vi "master_python_v2.0.vi"() -> ()   [LabVIEW 2026]
uses:
  <vilib>/Utility/error.llb/DialogType.ctl
  <vilib>/DAQmx/write.llb/DAQmx Write (Analog 2D DBL NChan NSamp).vi
  <vilib>/DAQmx/read.llb/DAQmx Read (Analog 1D Wfm NChan NSamp).vi
  <vilib>/DAQmx/miscellaneous.llb/DAQmx Fill In Error Info.vi
  <vilib>/Utility/inputDevices.llb/keyboardAcquire.vi
  Nanostage/Madlib.dll
panel:
  out "QPD":dbl
  out "Pos 0":dbl
  in  "Comment":string
  out "loop iteration":i32
  out "x start":dbl
  out "y start":dbl
  out "z start":dbl
  out "start iteration":dbl
  out "data":waveform(dbl)[](array[waveform])
  out "Numeric 2":i32
  out "Numeric":i32
  out "stop Ind":bool
  in  "Tab Control":enum32{"Main Control", "Calibration"}(tab)
  in  "Apply Force":bool
  out "Waveform Chart 6":waveform(dbl)(graph)
  out "Waveform Chart 5":waveform(dbl)(graph)
  in  "stop":bool
  in  "Record Data":bool
  in  "New File?":bool caption="new_file"
  out "QPD Position":cluster{"Array":dbl[], "Array":dbl[]}(graph)
  out "MT channels":waveform(dbl)[](graph)
  out "QPD Precise Position":cluster{"Array":dbl[], "Array":dbl[]}(graph)
  out "QPD Sum (Volt)":waveform(dbl)(graph)
  out "x":dbl
  out "y":dbl
  out "z":dbl
  in  "<":bool
  in  ">":bool
  in  "v":bool
  in  "^":bool
  in  "Down":bool
  in  "Up":bool
  in  "Fine":dbl=50.0
  in  "Step Size (nm)":bool
  in  "Course":dbl=500.0
  in  "Enable\ntapping":bool
  in  "DELAY (ms)":u32=10
  in  "x amplitude\n(um)":dbl
  in  "speed":i32=1
  in  "z amplitude (um)":dbl
  out "# oscillations":dbl
  in  "y amplitude\n(um)":dbl min=-25.0 max=25.0 step=0.05
  in  "Samples":u16=100 min=1 step=1
  in  "Centre":bool
  in  "Power Spectrum":bool
  in  "Duration (s)":dbl=2.0
  in  "Boolean":bool
  in  "Frequency":dbl=1.0 min=0.0 max=100.0 step=0.01
  in  "Amplitude":dbl=0.5 min=0.1 max=0.9 step=0.1
  in  "# Cycles":dbl=50.0 min=0.0 max=10000.0 step=0.001
  in  "Start Signal\nGen":bool
  in  "Desired Force (pN)":dbl step=0.01
  out "Measured Force (pN)":dbl(slide) scale=-2.0..2.0
  in  "Save Spectrum":bool
  in  "#":i32=1
  out "QPD nLR":waveform(dbl)(graph)
  out "QPD nBT":waveform(dbl)(graph)
  in  "Filename":path=path "C:/Users/localadmin/Desktop/220601 beadscan/7umscan2umbead.lvm"
  in  "Set 0 pN Position":bool
  out "QPD0":dbl
  in  "reinitialize?":bool
  in  "Conversion factor (pN/V)":dbl=1.0
  # "Left= anticlockwise"
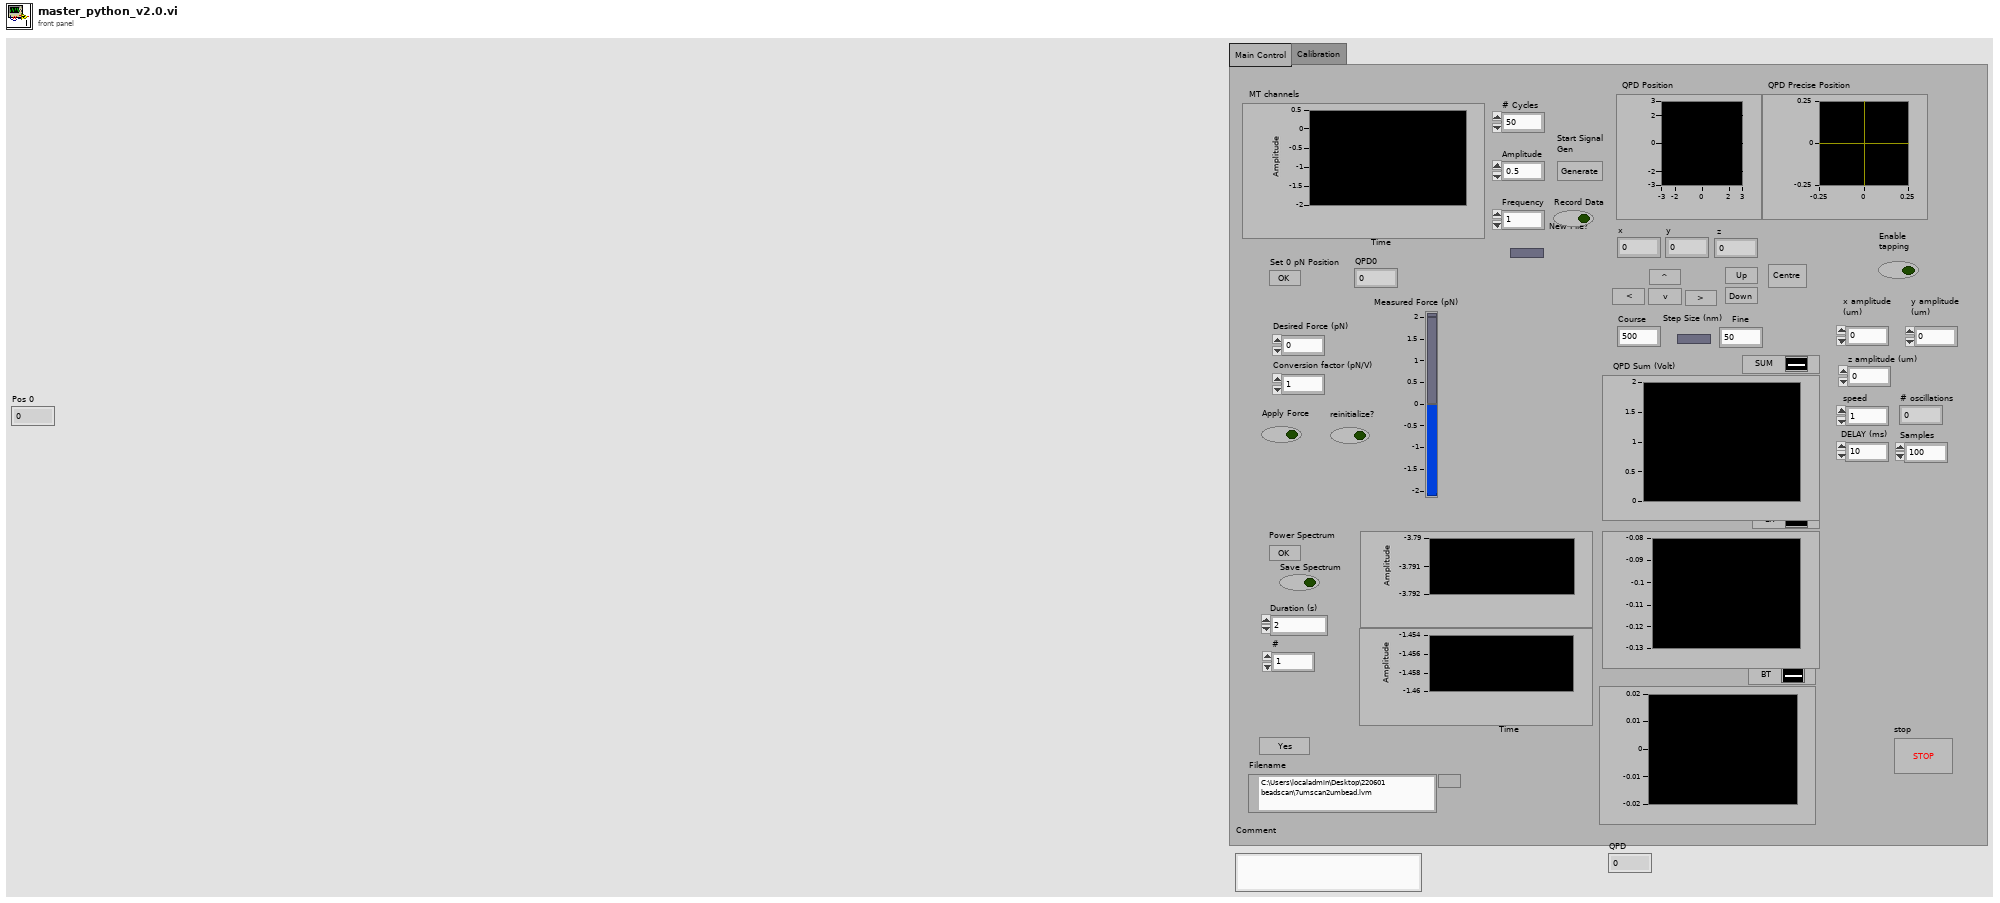
[diagram p1: front panel]
types:
  T1 = typedef "DialogType.ctl" = u16
  T2 = enum16{"Centre", "Move", "Tapping", "Calibration"}
  T3 = enum16{"0", "1", "2", "3", "4", "5", "6", "7", "8", "9", "A", "B", "C", "D", "E", "F", "G", "H", "I", "J", "K", "L", "M", "N", "O", "P", "Q", "R", "S", "T", "U", "V", "W", "X", "Y", "Z", "F1", "F2", "F3", "F4", "F5", "F6", "F7", "F8", "F9", "F10", "F11", "F12", "F13", "F14", "F15", "ADD", "BACK", "BACKSLASH", "CAPITAL", "COMMA", "DECIMAL", "DELETE", "DIVIDE", "DOWN", "END", "EQUALS", "ESCAPE", "GRAVE (`)", "HOME", "INSERT", "LBRACKET", "LCONTROL", "LEFT", "L ALT", "LSHIFT", "LWIN", "MINUS", "MULTIPLY", "NEXT", "NUMLOCK", "NUMPAD_0", "NUMPAD_1", "NUMPAD_2", "NUMPAD_3", "NUMPAD_4", "NUMPAD_5", "NUMPAD_6", "NUMPAD_7", "NUMPAD_8", "NUMPAD_9", "PAUSE", "PERIOD", "PRIOR (PG UP)", "RBRACKET", "RCONTROL", "RETURN", "RIGHT", "R ALT", "RSHIFT", "RWIN", "SCROLL", "SEMICOLON", "SLASH", "SPACE", "SUBTRACT", "TAB", "UP", "ENTER (num pad)", "' (quote)"}[]
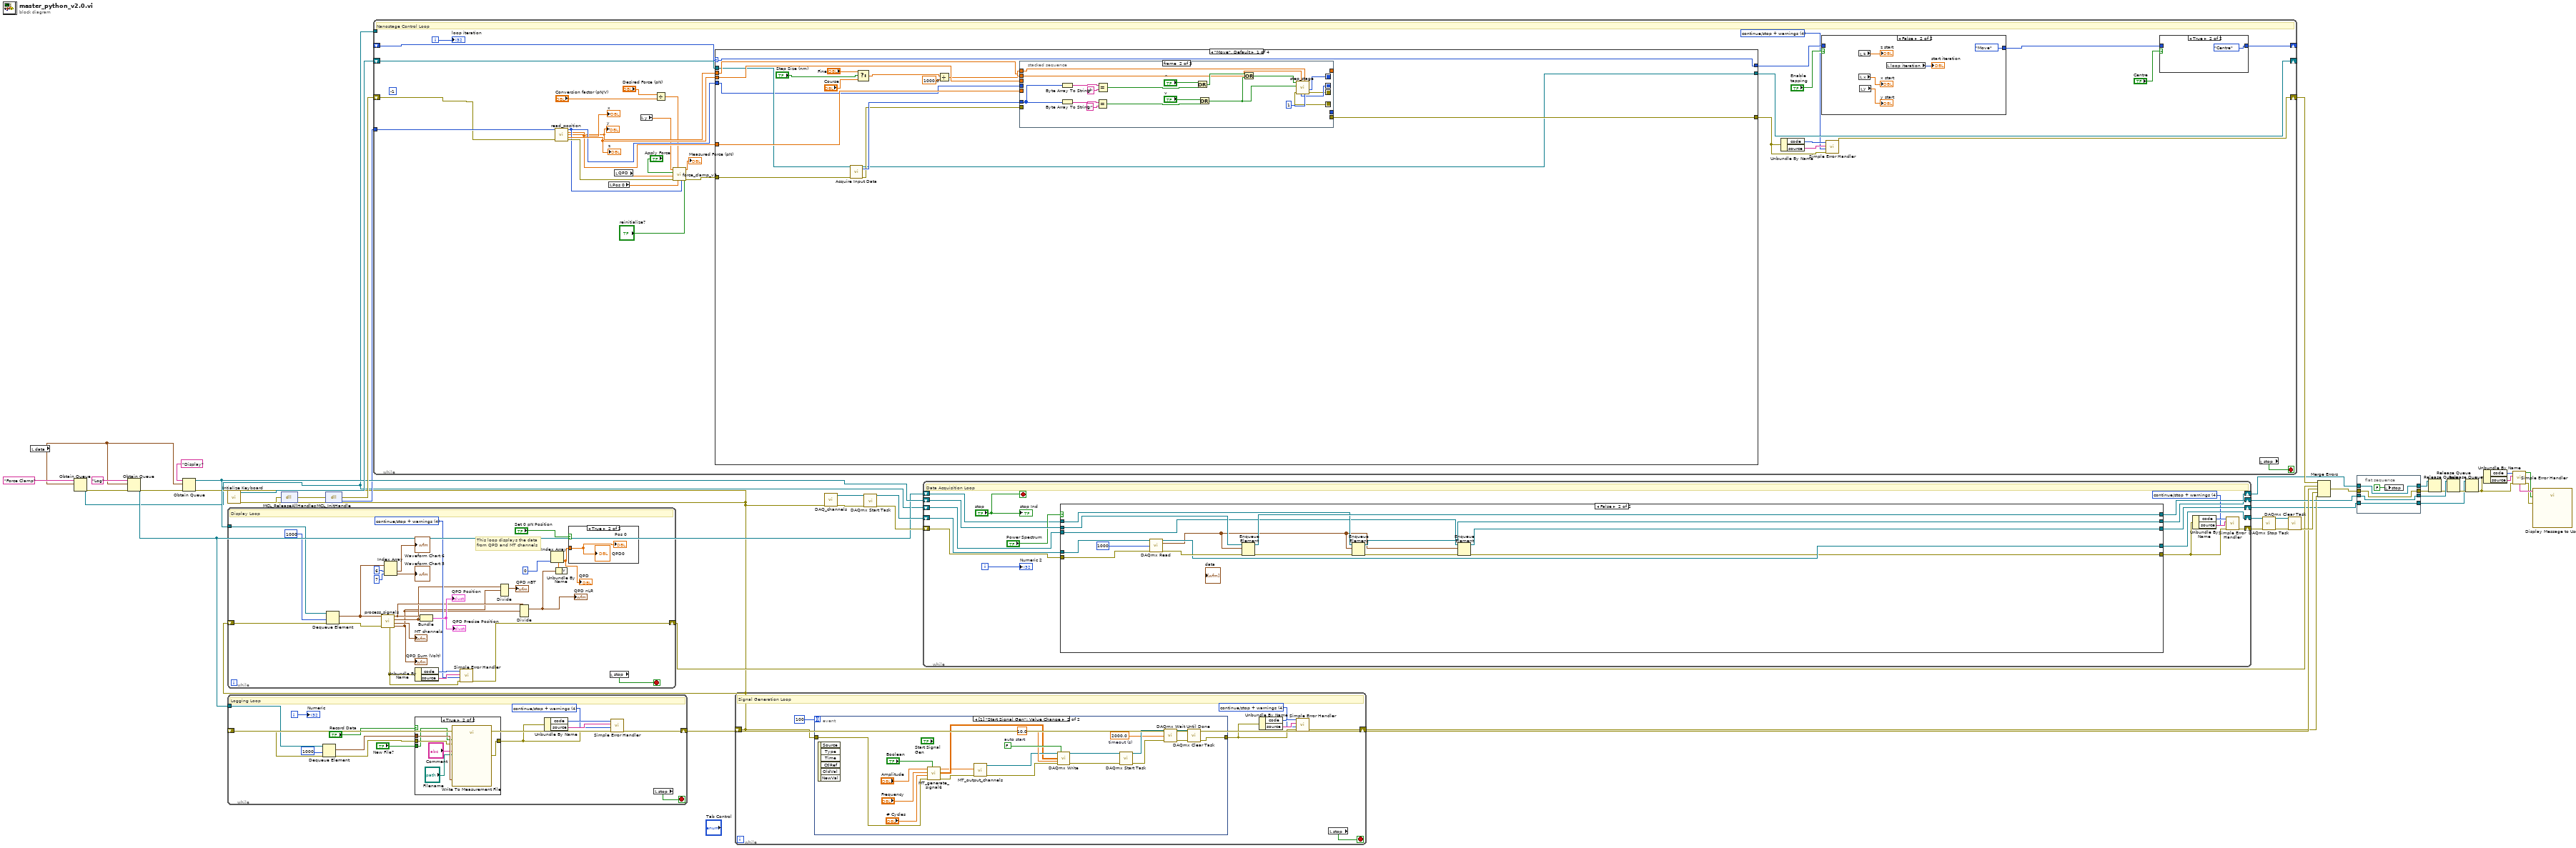
[diagram p0: block diagram]
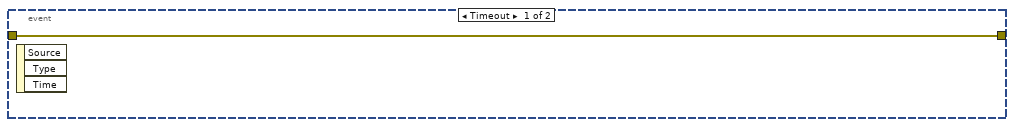
[diagram p2: hidden frame]
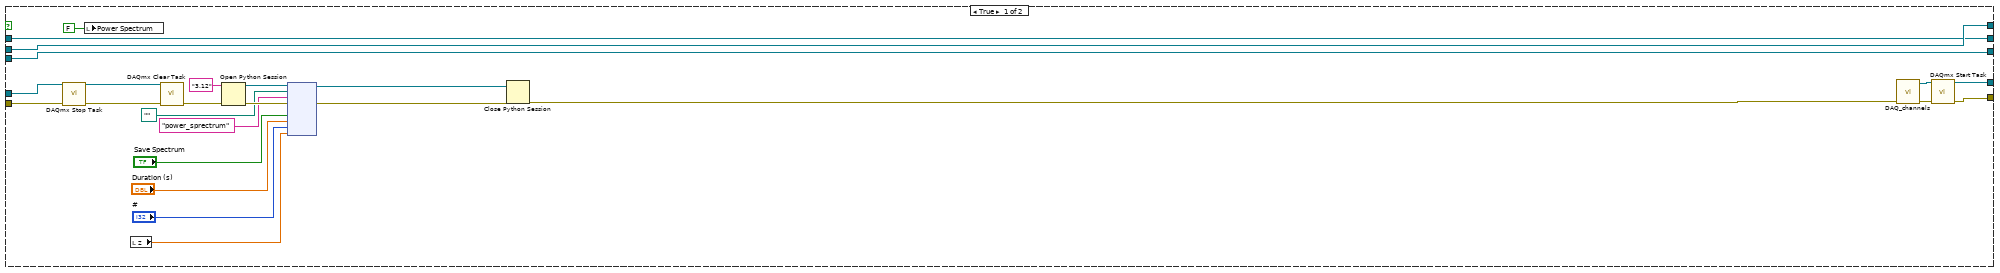
[diagram p3: hidden frame]
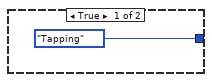
[diagram p6: hidden frame]
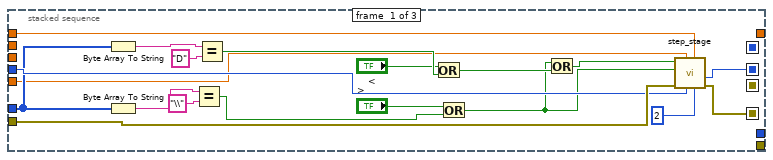
[diagram p7: hidden frame]
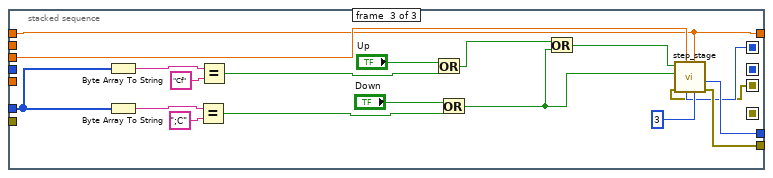
[diagram p8: hidden frame]
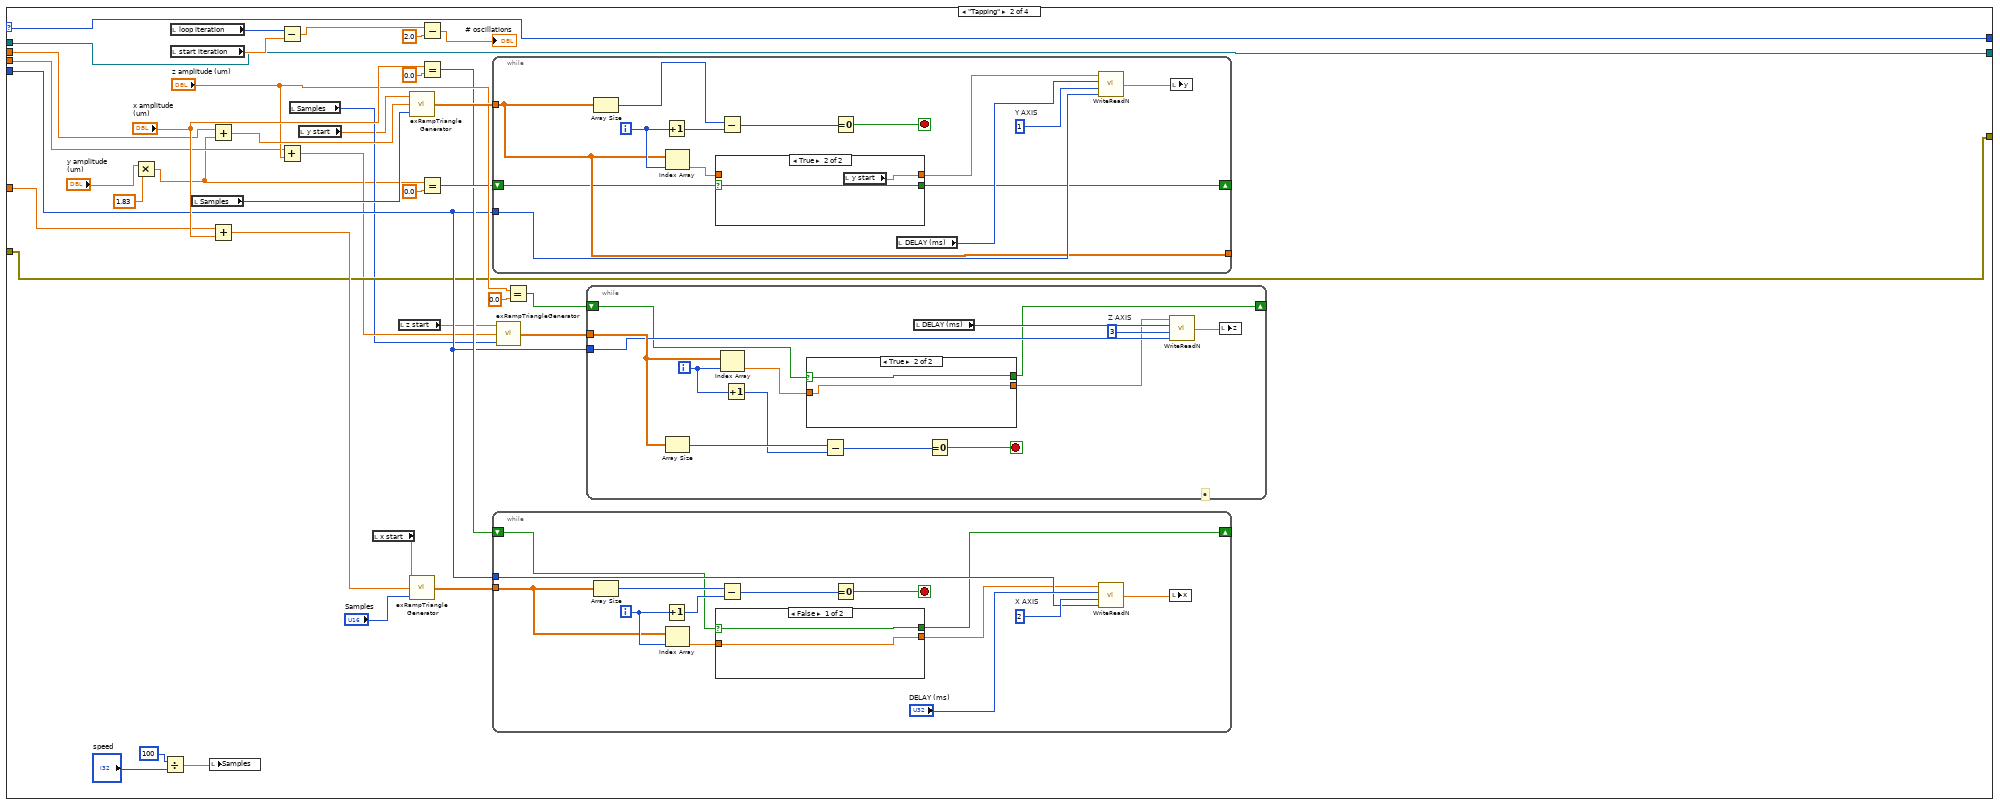
[diagram p9: hidden frame]
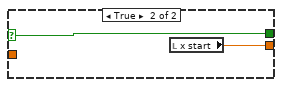
[diagram p12: hidden frame]
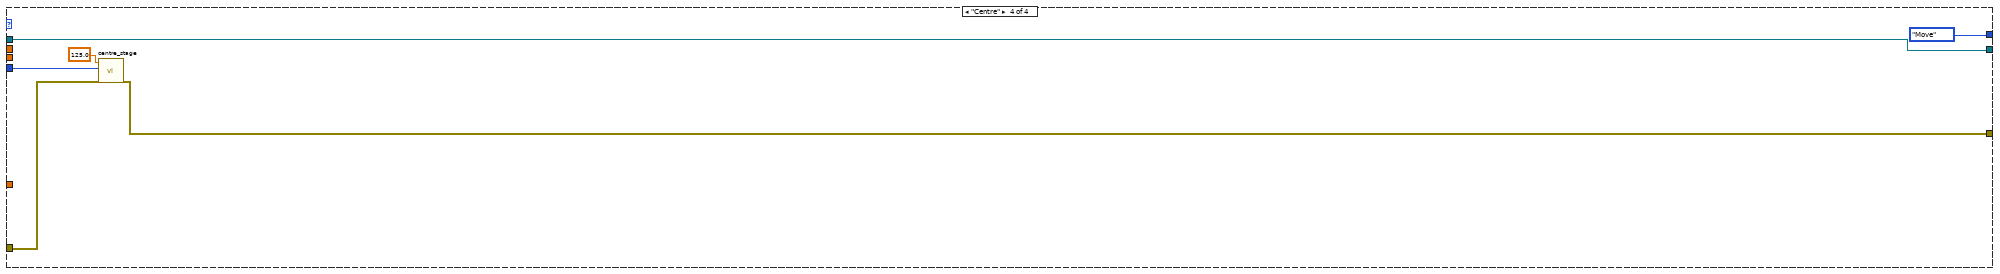
[diagram p14: hidden frame]
diagram:
  n1 = local read "data"() -> (w6:waveform(dbl)[])
  n2 = Obtain Queue(name (unnamed)="Force Clamp", element data type=w6) -> (queue out=w1:refnum<queue>, error out=w8:errorcluster)  [unwired: 3 in, 1 out]
  n3 = Obtain Queue(name (unnamed)="Log", element data type=w6, error in (no error)=w8) -> (queue out=w12:refnum<queue>, error out=w17:errorcluster)  [unwired: 2 in, 1 out]
  n4 = Obtain Queue(name (unnamed)="Display", element data type=w6, error in (no error)=w17) -> (queue out=w19:refnum<queue>, error out=w10:errorcluster)  [unwired: 2 in, 1 out]
  n5 = call <vilib>:"Intialize Keyboard.vi"("error in (no error)"=w10) -> ("error out"=w23:errorcluster, "device ID"=w21:refnum<k1>)  [unwired: 9 out]
  n6 = while {
    tunnel: w19 -> [w70]
    shift-right: [w55] -> w26
    shift-left: w10 -> [w69]
    stop <- w68 stop-if-true
    w54 = T1 4 items=["no dialog", "OK message", "continue or stop message", "OK message + warnings", "continue/stop + warnings"] ("type of dialog (OK msg:1)")
    # "This loop displays the data from QPD and MT channels"
    # "Display Loop"
    n7 = Dequeue Element(queue=w70, timeout in ms (-1)=1000, error in (no error)=w69) -> (element=w60:waveform(dbl)[], error out=w62:errorcluster)  [unwired: 2 out]
    n8 = call "process_signals.vi"("error in (no error)"=w62, "data"=w60) -> ("SUM"=w50:waveform(dbl), "MT"=→"MT channels":waveform(dbl)[], "BT"=w51:waveform(dbl), "LR"=w52:waveform(dbl), "error out"=w63:errorcluster)  [unwired: 5 in]
    "QPD Sum (Volt)" <- w50
    n9 = Index Array(array=w60, index #1=6 ("index"), index #2=7 ("index")) -> (element #1=→"Waveform Chart 6":waveform(dbl), element #2=→"Waveform Chart 5":waveform(dbl))
    n10 = Unbundle By Name(w63) -> ("code"=w65:i32, "source"=w64:string)
    n11 = Bundle("LR"=w52, "BT"=w51) -> (→"QPD Position" →"QPD Precise Position":cluster{"LR":waveform(dbl), "BT":waveform(dbl)})  [unwired: 1 in]
    n12 = call <vilib>:"Simple Error Handler.vi"("error code (no error:0)"=w65, "error source (\" \")"=w64, "type of dialog (OK msg:1)"=w54, "error in (no error)"=w63) -> ("error out"=w55:errorcluster)  [unwired: 1 in, 4 out]
    n13 = Divide(1:w50, 2:w51) -> (0:→"QPD nBT":waveform(dbl))  [unwired: 1 in, 1 out]
    n14 = Divide(1:w50, 2:w52) -> (0:w47:waveform(dbl))  [unwired: 1 in, 1 out]
    "QPD nLR" <- w47
    n15 = Unbundle By Name(w47) -> ("Y"=w48:dbl[])
    n16 = Index Array(array=w48, index=0) -> (element=w45:dbl)
    "QPD" <- w45
    n17 = case shown="True" "Set 0 pN Position" {
      tunnel: w45 -> [_ w71]
      frame False {
      }
      frame True {
        "Pos 0" <- w71
        "QPD0" <- w71
      }
    }
    n18 = local read "stop"() -> (w68:bool)
  }
  n19 = while {
    shift-right: [w73] -> w30
    shift-left: w10 -> [w85]
    tunnel: w12 -> [w84]
    i -> [w79]
    stop <- w74 stop-if-true
    w72 = T1 4 items=["no dialog", "OK message", "continue or stop message", "OK message + warnings", "continue/stop + warnings"] ("type of dialog (OK msg:1)")
    # "Logging Loop"
    n20 = Dequeue Element(queue=w84, timeout in ms (-1)=1000, error in (no error)=w85) -> (element=w81:waveform(dbl)[], error out=w82:errorcluster)  [unwired: 2 out]
    n21 = case shown="True" "Record Data" {
      tunnel: [w86 w92] -> w75
      tunnel: w81 -> [_ w91]
      tunnel: "New File?" -> [_ w88]
      tunnel: w82 -> [w86 w90]
      frame False {
      }
      frame True {
        n22 = call "Write To Measurement File"("Signals"=w91, "new_file"=w88, "error in (no error)"=w90, "Filename"="Filename", "Comment"="Comment") -> ("error out"=w92:errorcluster)  [unwired: 12 in, 2 out]
      }
    }
    n23 = Unbundle By Name(w75) -> ("code"=w77:i32, "source"=w76:string)
    n24 = call <vilib>:"Simple Error Handler.vi"("error code (no error:0)"=w77, "error source (\" \")"=w76, "type of dialog (OK msg:1)"=w72, "error in (no error)"=w75) -> ("error out"=w73:errorcluster)  [unwired: 1 in, 4 out]
    n25 = local read "stop"() -> (w74:bool)
    "Numeric" <- w79
  }
  n26 = dll-call lib="C:/Users/psmr500/PycharmProjects/COMBI-Tweez/LabVIEW Microscope Control/Nanostage/MADLib.dll" fn="MCL_ReleaseAllHandles"(error in=w23) -> (error out=w24:errorcluster)  [unwired: 3 in, 1 out]
  n27 = dll-call lib="C:/Users/psmr500/PycharmProjects/COMBI-Tweez/LabVIEW Microscope Control/Nanostage/MADLib.dll" fn="MCL_InitHandle"(error in=w24) -> (error out=w22:errorcluster, "return type"=w11:i32)  [unwired: 2 in, 1 out]
  n28 = while {
    shift-right: [w106] -> w20
    shift-left: w22 -> [w101]
    shift-right: [w117] -> _
    shift-left: w21 -> [w119]
    shift-right: [w111] -> _
    shift-left: _ -> [w118]
    tunnel: w11 -> [w116]
    tunnel: w1 -> [_]
    i -> [w114]
    stop <- w124 stop-if-true
    (unwired) -1 ("timeout in ms (-1)")
    w105 = T1 4 items=["no dialog", "OK message", "continue or stop message", "OK message + warnings", "continue/stop + warnings"] ("type of dialog (OK msg:1)")
    # "Nanostage Control Loop"
    n29 = call "read_position.vi"("handle in"=w116, "error in (no error)"=w101) -> ("handle out"=w107:i32, "x"=w104:dbl, "y"=w103:dbl, "z"=w120:dbl, "error out"=w109:errorcluster)  [unwired: 9 in]
    "x" <- w104
    "y" <- w103
    "z" <- w120
    n30 = local read "Pos 0"() -> (w98:dbl)
    n31 = local read "QPD"() -> (w99:dbl)
    n32 = local read "y"() -> (w100:dbl)
    n33 = Divide(x="Desired Force (pN)", y="Conversion factor (pN/V)") -> (x/y=w95:dbl)
    n34 = call "force_clamp_v3.vi"("reinitialize? (F) 2"="reinitialize?", "handle in"=w107, "Pos 0"=w98, "Desired Force (pN)"=w95, "error in (no error)"=w109, "QPD"=w99, "Apply Force"="Apply Force", "Nanostage"=w100) -> ("error out"=w108:errorcluster, "QPD delta"=→"Measured Force (pN)":dbl)  [unwired: 2 in]
    n35 = case shown="\"Move\", Default" w118 {
      selector: w118 -> [w133 w217 w308 _]
      tunnel: w108 -> [w139 w219 w306 w323]
      tunnel: w107 -> [w137 w220 w307 w322]
      tunnel: [w135 w219 w300 w321] -> w121
      tunnel: w104 -> [w149 w222 w310 _]
      tunnel: w103 -> [w148 w221 w309 _]
      tunnel: w120 -> [w147 w216 _ _]
      tunnel: w119 -> [w140 w218 w299 w318]
      tunnel: [w133 w217 w308 T2."Move"] -> w115
      tunnel: [w134 w218 w299 w318] -> w117
      frame "Move", Default {
        n36 = call-poly <vilib>:"Acquire Input Data.vi"("device ID"=w140, "error in (no error)"=w139) -> ("device ID"=w134:refnum<k1>, "keys pressed"=w138:T3, "error out"=w136:errorcluster)  [unwired: 15 out]
        n37 = Select(t="Fine", s="Step Size (nm)", f="Course") -> (s? t:f=w143:dbl)
        n38 = Divide(x=w143, y=1000.0) -> (x/y=w141:dbl)
        n39 = stacked-sequence {
          seq-local: [w165 _ _] -> [_ w185 _]
          seq-local: [w164 _ _] -> [_ w184 _]
          seq-local: [_ w182 _] -> [_ _ w202]
          seq-local: [_ w183 _] -> [_ _ w201]
          tunnel: w136 -> [w168 _ _]
          tunnel: w137 -> [w167 _ _]
          tunnel: w149 -> [w151 _ _]
          tunnel: w148 -> [_ w169 _]
          tunnel: w147 -> [_ _ w205]
          tunnel: [_ _ w203] -> w135
          tunnel: [_ _ w204] -> _
          tunnel: w138 -> [w153 w171 w189]
          tunnel: [_ _ w188] -> _
          tunnel: w141 -> [w152 w170 w188]
          frame #0 {
            n40 = Byte Array To String(unsigned byte array=w153) -> (string=w161:string)
            n41 = Byte Array To String(unsigned byte array=w153) -> (string=w163:string)
            n42 = Equal?(x=w163, y="\\") -> (x = y?=w159:bool)
            n43 = Equal?(x=w161, y="D") -> (x = y?=w158:bool)
            n44 = Or(x="<", y=w158) -> (x .or. y?=w155:bool)
            n45 = Or(x=">", y=w159) -> (x .or. y?=w150:bool)
            n46 = Or(x=w150, y=w155) -> (x .or. y?=w154:bool)
            n47 = call "step_stage.vi"("axis"=u32 2, "step"=w152, "handle"=w167, "position"=w151, "error in"=w168, "+/-"=w150, "move"=w154) -> ("error out"=w164:errorcluster, "handle out"=w165:i32)  [unwired: 3 in]
          }
          frame #1 {
            n48 = Byte Array To String(unsigned byte array=w171) -> (string=w181:string)
            n49 = Byte Array To String(unsigned byte array=w171) -> (string=w179:string)
            n50 = Equal?(x=w179, y=";") -> (x = y?=w174:bool)
            n51 = Equal?(x=w181, y="f") -> (x = y?=w177:bool)
            n52 = Or(x="^", y=w177) -> (x .or. y?=w173:bool)
            n53 = Or(x="v", y=w174) -> (x .or. y?=w172:bool)
            n54 = Or(x=w173, y=w172) -> (x .or. y?=w187:bool)
            n55 = call "step_stage.vi"("axis"=u32 1, "step"=w170, "handle"=w185, "position"=w169, "error in"=w184, "+/-"=w172, "move"=w187) -> ("error out"=w183:errorcluster, "handle out"=w182:i32)  [unwired: 3 in]
          }
          frame #2 {
            n56 = Byte Array To String(unsigned byte array=w189) -> (string=w200:string)
            n57 = Byte Array To String(unsigned byte array=w189) -> (string=w198:string)
            n58 = Equal?(x=w198, y=";C") -> (x = y?=w195:bool)
            n59 = Equal?(x=w200, y="Cf") -> (x = y?=w196:bool)
            n60 = Or(x="Up", y=w196) -> (x .or. y?=w194:bool)
            n61 = Or(x="Down", y=w195) -> (x .or. y?=w192:bool)
            n62 = Or(x=w194, y=w192) -> (x .or. y?=w193:bool)
            n63 = call "step_stage.vi"("axis"=u32 3, "step"=w188, "handle"=w202, "position"=w205, "error in"=w201, "+/-"=w192, "move"=w193) -> ("error out"=w203:errorcluster, "handle out"=w204:i32)  [unwired: 3 in]
          }
        }
      }
      frame "Tapping" {
        n64 = Multiply(x="y amplitude\n(um)", y=1.83) -> (x*y=w208:dbl)
        n65 = Divide(x=100, y="speed") -> (x/y=w239:dbl)
        n66 = local read "loop iteration"() -> (w234:i32)
        n67 = local read "start iteration"() -> (w235:dbl)
        n68 = local read "Samples"() -> (w236:u16)
        n69 = local write "Samples"(w239) -> ()
        n70 = Add(x=w221, y=w208) -> (x+y=w238:dbl)
        n71 = Add(x=w222, y="x amplitude\n(um)") -> (x+y=w243:dbl)
        n72 = Subtract(x=w234, y=w235) -> (x-y=w233:dbl)
        n73 = Add(x=w216, y="z amplitude (um)") -> (x+y=w215:dbl)
        n74 = local read "Samples"() -> (w214:u16)
        n75 = local read "y start"() -> (w210:dbl)
        n76 = local read "x start"() -> (w212:dbl)
        n77 = local read "z start"() -> (w211:dbl)
        n78 = call "exRampTriangleGenerator.vi"("Number of positions"=w236, "End(um)"=w238, "Start(um)"=w210) -> ("Array"=w237:dbl[])
        n79 = call "exRampTriangleGenerator.vi"("Number of positions"="Samples", "End(um)"=w243, "Start(um)"=w212) -> ("Array"=w244:dbl[])
        n80 = Subtract(x=w233, y=2.0) -> (x-y=→"# oscillations":dbl)
        n81 = Equal?(x="x amplitude\n(um)", y=0.0) -> (x = y?=w224:bool)
        n82 = Equal?(x=w208, y=0.0) -> (x = y?=w225:bool)
        n83 = while {
          tunnel: [w268] -> _
          tunnel: w220 -> [w275]
          tunnel: w237 -> [w268]
          shift-right: [w264] -> _
          shift-left: w225 -> [w265]
          i -> [w276]
          stop <- w270 stop-if-true
          w271 = 1  # Y AXIS
          n84 = Array Size(array=w268) -> (size(s)=w273:i32)
          n85 = Increment(x=w276) -> (x+1=w272:i32)
          n86 = Index Array(array=w268, index=w276) -> (element=w267:dbl)
          n87 = case shown="True" w265 {
            selector: w265 -> [w277 w280]
            tunnel: w267 -> [w278 _]
            tunnel: [w278 w279] -> w266
            tunnel: [w277 w280] -> w264
            frame False {
            }
            frame True {
              n88 = local read "y start"() -> (w279:dbl)
            }
          }
          n89 = Subtract(x=w273, y=w272) -> (x-y=w274:i32)
          n90 = Equal To 0?(x=w274) -> (x = 0?=w270:bool)
          n91 = local read "DELAY (ms)"() -> (w269:u32)
          n92 = call "WriteReadN.vi"("Handle"=w275, "Axis"=w271, "Delay (ms)"=w269, "Move to (um)"=w266) -> ("Current Position (um)"=w263:dbl)
          n93 = local write "y"(w263) -> ()
        }
        n94 = while {
          tunnel: w244 -> [w286]
          tunnel: w220 -> [w287]
          shift-right: [w282] -> _
          shift-left: w224 -> [w283]
          i -> [w290]
          stop <- w292 stop-if-true
          w288 = 2  # X AXIS
          n95 = Array Size(array=w286) -> (size(s)=w293:i32)
          n96 = Increment(x=w290) -> (x+1=w291:i32)
          n97 = Index Array(array=w286, index=w290) -> (element=w285:dbl)
          n98 = case shown="False" w283 {
            selector: w283 -> [w295 w298]
            tunnel: w285 -> [w296 _]
            tunnel: [w296 w297] -> w284
            tunnel: [w295 w298] -> w282
            frame False {
            }
            frame True {
              n99 = local read "x start"() -> (w297:dbl)
            }
          }
          n100 = Subtract(x=w293, y=w291) -> (x-y=w294:i32)
          n101 = Equal To 0?(x=w294) -> (x = 0?=w292:bool)
          n102 = call "WriteReadN.vi"("Handle"=w287, "Axis"=w288, "Delay (ms)"="DELAY (ms)", "Move to (um)"=w284) -> ("Current Position (um)"=w281:dbl)
          n103 = local write "x"(w281) -> ()
        }
        n104 = call "exRampTriangleGenerator.vi"("Number of positions"=w214, "End(um)"=w215, "Start(um)"=w211) -> ("Array"=w213:dbl[])
        n105 = Equal?(x="z amplitude (um)", y=0.0) -> (x = y?=w223:bool)
        n106 = while {
          tunnel: w213 -> [w251]
          tunnel: w220 -> [w250]
          shift-right: [w246] -> _
          shift-left: w223 -> [w247]
          i -> [w254]
          stop <- w256 stop-if-true
          w253 = 3  # Z AXIS
          # "e"
          n107 = Array Size(array=w251) -> (size(s)=w257:i32)
          n108 = Index Array(array=w251, index=w254) -> (element=w249:dbl)
          n109 = Increment(x=w254) -> (x+1=w255:i32)
          n110 = case shown="True" w247 {
            selector: w247 -> [w259 w262]
            tunnel: w249 -> [w260 w261]
            tunnel: [w260 w261] -> w248
            tunnel: [w259 w262] -> w246
            frame False {
            }
            frame True {
            }
          }
          n111 = Subtract(x=w257, y=w255) -> (x-y=w258:i32)
          n112 = local read "DELAY (ms)"() -> (w252:u32)
          n113 = Equal To 0?(x=w258) -> (x = 0?=w256:bool)
          n114 = call "WriteReadN.vi"("Handle"=w250, "Axis"=w253, "Delay (ms)"=w252, "Move to (um)"=w248) -> ("Current Position (um)"=w245:dbl)
          n115 = local write "z"(w245) -> ()
        }
      }
      frame "Calibration" {
        n116 = flat-sequence {
          tunnel: w306 -> [w311]
          tunnel: [w311] -> w301
          tunnel: [w312] -> w302
          tunnel: w301 -> [w312]
          tunnel: w307 -> [_]
          tunnel: w310 -> [_]
          tunnel: w309 -> [_]
          tunnel: [w313] -> w303
          tunnel: w302 -> [w313]
          tunnel: [w314] -> w304
          tunnel: w303 -> [w314]
          tunnel: [w316] -> _
          tunnel: w307 -> [w316]
          tunnel: [w315] -> w305
          tunnel: w304 -> [w315]
          tunnel: w305 -> [w317]
          tunnel: [w317] -> w300
          frame #0 {
          }
          frame #1 {
          }
          frame #2 {
          }
          frame #3 {
          }
          frame #4 {
          }
          frame #5 {
          }
        }
      }
      frame "Centre" {
        n117 = call "centre_stage.vi"("error in"=w323, "handle in"=w322, "Destination"=125.0) -> ("error out"=w321:errorcluster)  [unwired: 7 in, 1 out]
      }
    }
    n118 = Unbundle By Name(w121) -> ("code"=w123:i32, "source"=w122:string)
    n119 = case shown="False" "Enable\ntapping" {
      tunnel: w115 -> [_ _]
      tunnel: [T2."Tapping" T2."Move"] -> w102
      frame True {
      }
      frame False {
        n120 = local read "z"() -> (→"z start":dbl)
        n121 = local read "x"() -> (→"x start":dbl)
        n122 = local read "y"() -> (→"y start":dbl)
        n123 = local read "loop iteration"() -> (→"start iteration":i32)
      }
    }
    n124 = call <vilib>:"Simple Error Handler.vi"("error code (no error:0)"=w123, "error source (\" \")"=w122, "type of dialog (OK msg:1)"=w105, "error in (no error)"=w121) -> ("error out"=w106:errorcluster)  [unwired: 1 in, 4 out]
    n125 = case shown="True" "Centre" {
      tunnel: [w125 T2."Centre"] -> w111
      tunnel: w102 -> [w125 _]
      frame False {
      }
      frame True {
      }
    }
    n126 = local read "stop"() -> (w124:bool)
    "loop iteration" <- w114
  }
  n127 = while {
    shift-right: [w325] -> w9
    shift-left: w10 -> [w330]
    stop <- w331 stop-if-true
    w326 = T1 4 items=["no dialog", "OK message", "continue or stop message", "OK message + warnings", "continue/stop + warnings"] ("type of dialog (OK msg:1)")
    # "Signal Generation Loop"
    n128 = event shown="[1] \"Start Signal Gen\": Value Change" {
      selector: _ -> [_ _]
      dyn-events: _ -> [_ _]
      timeout: 100 -> [_ _]
      tunnel: [w332 w335] -> w324
      tunnel: w330 -> [w332 w334]
      event Timeout {
        n129 = event-data() -> ()  [unwired: 1 in, 3 out]
      }
      event "Start Signal\nGen": Value Change {
        w344 = 2000.0  # timeout (s)
        w343 = FALSE  # auto start
        n130 = event-data() -> ()  [unwired: 1 in, 6 out]
        n131 = call "MT_generate_signal6.vi"("Direction"="Boolean", "error in (no error)"=w334, "# cycles"="# Cycles", "frequency"="Frequency", "amplitude"="Amplitude") -> ("error out"=w340:errorcluster, "signals out"=w338:dbl[][], "# samples"=w337:dbl)  [unwired: 4 in]
        n132 = call "MT_output_channels.vi"("error in"=w340, "number of samples"=w337) -> ("error out"=w339:errorcluster, "task out"=w341:refnum<k21>)  [unwired: 8 in]
        n133 = call-poly <vilib>:"DAQmx Write.vi"("task/channels in"=w341, "auto start"=w343, "data"=w338, "timeout"=10.0, "error in"=w339) -> ("task out"=w348:refnum<k21>, "error out"=w349:errorcluster)  [unwired: 8 in, 1 out]
        n134 = call <vilib>:"DAQmx Start Task.vi"("task/channels in"=w348, "error in"=w349) -> ("task out"=w345:refnum<k21>, "error out"=w346:errorcluster)  [unwired: 12 in]
        n135 = call <vilib>:"DAQmx Wait Until Done.vi"("task/channels in"=w345, "timeout (sec)"=w344, "error in"=w346) -> ("task out"=w350:refnum<k21>, "error out"=w347:errorcluster)  [unwired: 11 in]
        n136 = call <vilib>:"DAQmx Clear Task.vi"("task in"=w350, "error in"=w347) -> ("error out"=w335:errorcluster)  [unwired: 13 in]
      }
    }
    n137 = Unbundle By Name(w324) -> ("code"=w328:i32, "source"=w327:string)
    n138 = call <vilib>:"Simple Error Handler.vi"("error code (no error:0)"=w328, "error source (\" \")"=w327, "type of dialog (OK msg:1)"=w326, "error in (no error)"=w324) -> ("error out"=w325:errorcluster)  [unwired: 1 in, 4 out]
    n139 = local read "stop"() -> (w331:bool)
  }
  n140 = call "DAQ_channels.vi"("error in"=w10) -> ("error out"=w38:errorcluster, "task out"=w39:refnum<k21>)  [unwired: 9 in]
  n141 = call <vilib>:"DAQmx Start Task.vi"("task/channels in"=w39, "error in"=w38) -> ("task out"=w42:refnum<k21>, "error out"=w43:errorcluster)  [unwired: 12 in]
  n142 = while {
    shift-right: [w354] -> w37
    shift-left: w43 -> [w369]
    shift-right: [w366] -> w29
    shift-left: w19 -> [w367]
    shift-right: [w363] -> w25
    shift-left: w42 -> [w368]
    shift-right: [w358] -> w16
    shift-left: w12 -> [w357]
    shift-right: [w355] -> w2
    shift-left: w1 -> [w356]
    i -> [w364]
    stop <- "stop" stop-if-true
    w353 = T1 4 items=["no dialog", "OK message", "continue or stop message", "OK message + warnings", "continue/stop + warnings"] ("type of dialog (OK msg:1)")
    # "Data Acquisition Loop"
    n143 = case shown="False" "Power Spectrum" {
      tunnel: w369 -> [w393 w409]
      tunnel: w368 -> [w394 w407]
      tunnel: w367 -> [w392 w406]
      tunnel: [w392 w405] -> w366
      tunnel: [w385 w404] -> w363
      tunnel: [w384 w398] -> w359
      tunnel: w357 -> [w391 w402]
      tunnel: [w391 w400] -> w358
      tunnel: w356 -> [w383 w397]
      tunnel: [w383 w396] -> w355
      frame True {
        n144 = call <vilib>:"DAQmx Stop Task.vi"("task/channels in"=w394, "error in"=w393) -> ("task out"=w390:refnum<k21>, "error out"=w389:errorcluster)  [unwired: 12 in]
        n145 = local write "Power Spectrum"(FALSE ("Power Spectrum")) -> ()
        n146 = local read "z"() -> (w373:dbl)
        n147 = call <vilib>:"DAQmx Clear Task.vi"("task in"=w390, "error in"=w389) -> ("error out"=w381:errorcluster)  [unwired: 13 in]
        n148 = Open Python Session(python version="3.12" ("Python version"), 3:w381) -> (session out=w379:refnum<k35>, error out=w380:errorcluster)  [unwired: 1 in]
        n149 = node(w379, path "" ("module path"), "power_sprectrum" ("function name"), w380, "Save Spectrum", "Duration (s)", "#", w373) -> (w372:refnum<k35>, w371:errorcluster)  [unwired: 6 in, 2 out]
        n150 = Close Python Session(session in=w372, error in=w371) -> (11:w370:errorcluster)
        n151 = call "DAQ_channels.vi"("error in"=w370) -> ("error out"=w386:errorcluster, "task out"=w387:refnum<k21>)  [unwired: 9 in]
        n152 = call <vilib>:"DAQmx Start Task.vi"("task/channels in"=w387, "error in"=w386) -> ("task out"=w385:refnum<k21>, "error out"=w384:errorcluster)  [unwired: 12 in]
      }
      frame False {
        n153 = call-poly <vilib>:"DAQmx Read.vi"("task/channels in"=w407, "number of samples per channel"=1000, "error in"=w409) -> ("task out"=w404:refnum<k21>, "data"=w395:waveform(dbl)[], "error out"=w408:errorcluster)  [unwired: 10 in]
        n154 = Enqueue Element(queue=w406, element=w395, error in (no error)=w408) -> (queue out=w405:refnum<queue>, error out=w401:errorcluster)  [unwired: 2 out]
        n155 = Enqueue Element(queue=w402, element=w395, error in (no error)=w401) -> (queue out=w400:refnum<queue>, error out=w399:errorcluster)  [unwired: 2 out]
        n156 = Enqueue Element(queue=w397, element=w395, error in (no error)=w399) -> (queue out=w396:refnum<queue>, error out=w398:errorcluster)  [unwired: 2 out]
      }
    }
    n157 = Unbundle By Name(w359) -> ("code"=w361:i32, "source"=w360:string)
    n158 = call <vilib>:"Simple Error Handler.vi"("error code (no error:0)"=w361, "error source (\" \")"=w360, "type of dialog (OK msg:1)"=w353, "error in (no error)"=w359) -> ("error out"=w354:errorcluster)  [unwired: 1 in, 4 out]
    "Numeric 2" <- w364
    "stop Ind" <- "stop"
  }
  n159 = call <vilib>:"DAQmx Stop Task.vi"("task/channels in"=w25, "error in"=w37) -> ("task out"=w35:refnum<k21>, "error out"=w36:errorcluster)  [unwired: 12 in]
  n160 = call <vilib>:"DAQmx Clear Task.vi"("task in"=w35, "error in"=w36) -> ("error out"=w31:errorcluster)  [unwired: 13 in]
  n161 = Merge Errors(w20, w26, w30, w31, w9) -> (w27:errorcluster)
  n162 = flat-sequence {
    tunnel: w29 -> [w414]
    tunnel: [w414] -> w28
    tunnel: w27 -> [w413]
    tunnel: [w413] -> w14
    tunnel: w16 -> [w411]
    tunnel: [w411] -> w15
    tunnel: [w410] -> w3
    tunnel: w2 -> [w410]
    frame #0 {
      n163 = local write "stop"(FALSE ("create if not found? (T)")) -> ()
    }
  }
  n164 = Release Queue(queue=w15, error in (no error)=w14) -> (error out=w13:errorcluster)  [unwired: 1 in, 2 out]
  n165 = Release Queue(queue=w28, error in (no error)=w13) -> (error out=w5:errorcluster)  [unwired: 1 in, 2 out]
  n166 = Release Queue(queue=w3, error in (no error)=w5) -> (error out=w4:errorcluster)  [unwired: 1 in, 2 out]
  n167 = Unbundle By Name(w4) -> ("code"=w41:i32, "source"=w40:string)
  n168 = call <vilib>:"Simple Error Handler.vi"("error code (no error:0)"=w41, "error source (\" \")"=w40, "error in (no error)"=w4) -> ("error?"=w32:bool, "error out"=w33:errorcluster, "message"=w34:string)  [unwired: 2 in, 2 out]
  n169 = call "Display Message to User"("error in (no error)"=w33, "Enable"=w32, "Message"=w34) -> ()  [unwired: 7 in, 2 out]
